vi "cblas zher2.vi"(0 "x":cdb[](array[numeric]), 1 "y":cdb[](array[numeric]), 2 "A":T2, 3 "alpha":cdb=1.0+0.0i, 5 "order":T3=101 items=["CblasRowMajor"=101, "CblasColMajor"=102], 7 "uplo":T1=121 items=["CblasUpper"=121, "CblasLower"=122], 8 "lda":i32, 10 "incx":i32=1, 11 "n":i32=-1, 12 "incy":i32=1) -> (14 "zher2":T2, 19 "error":i32)   [LabVIEW 2024, in "NI_AALBLAS.lvlib"]
uses:
  NI_AALBLAS.lvlib
  ComplexMatrix.ctl
  Order.ctl
  UpLo.ctl
  <resource>/lvblas.dll
  NI_Matrix.lvlib
panel:
  # "void cblas_zher2(order, uplo, n, *alpha, *x, incx, *y, incy, *A, lda)"
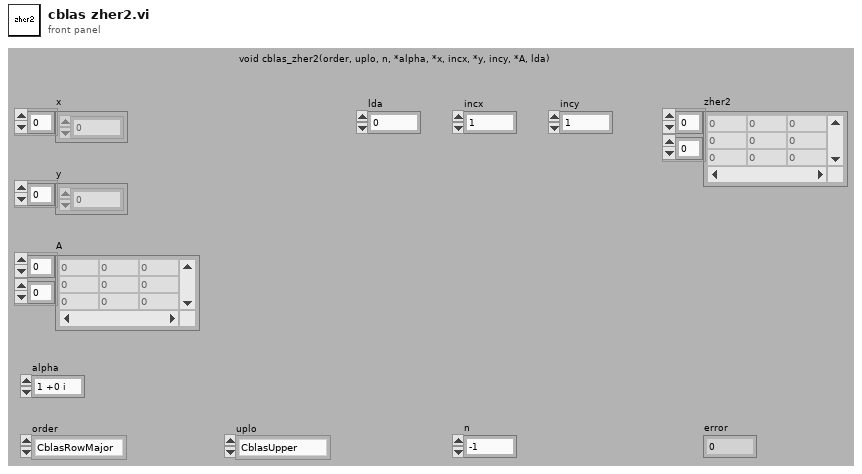
[diagram p1: front panel]
types:
  T1 = typedef "NI_AALBLAS.lvlib/UpLo.ctl" = i32
  T2 = typedef "NI_Matrix.lvlib/ComplexMatrix.ctl" = cdb[][]
  T3 = typedef "NI_AALBLAS.lvlib/Order.ctl" = i32
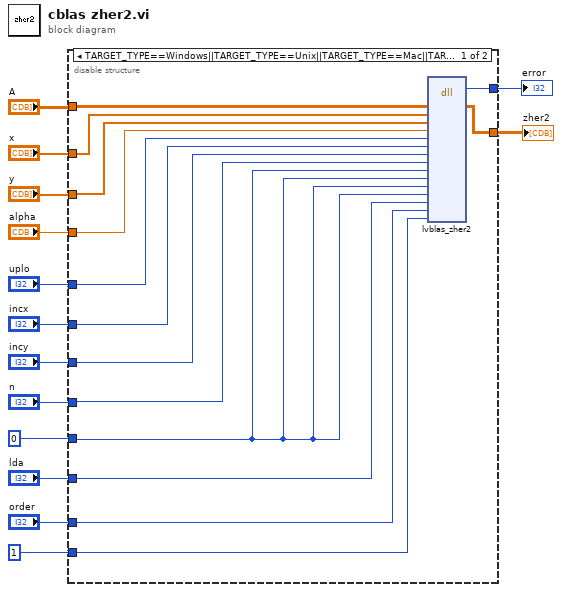
[diagram p0: block diagram]
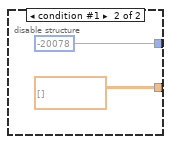
[diagram p2: hidden frame]
diagram:
  n1 = disable-structure shown="TARGET_TYPE==Windows||TARGET_TYPE==Unix||TARGET_TYPE==Mac||TARGET_TYPE==RT" {
    disable-tunnel: "x" -> [w25 _]
    disable-tunnel: "A" -> [w26 _]
    disable-tunnel: [w28 -20078 ("error")] -> w7
    disable-tunnel: 0 -> [w20 _]
    disable-tunnel: "lda" -> [w19 _]
    disable-tunnel: [w27 T2 [] ("Complex Matrix")] -> w8
    disable-tunnel: "uplo" -> [w22 _]
    disable-tunnel: "n" -> [w21 _]
    disable-tunnel: "alpha" -> [w23 _]
    disable-tunnel: "y" -> [w24 _]
    disable-tunnel: "order" -> [w18 _]
    disable-tunnel: "incx" -> [w17 _]
    disable-tunnel: "incy" -> [w16 _]
    disable-tunnel: 1 -> [w15 _]
    frame condition #0 (active) {
      n2 = dll-call lib="C:/Program Files (x86)/National Instruments/LabVIEW 2024/resource/lvblas.*" fn="lvblas_zher2" ("CBLAS.dll:MtrxxVectH")("a"=w26, "x"=w25, "y"=w24, "alpha"=w23, "uplo"=w22, "IncX"=w17, "IncY"=w16, "n"=w21, "startARow"=w20, "startACol"=w20, "startX"=w20, "startY"=w20, "lda"=w19, "order"=w18, "check"=w15) -> ("error"=w28:i32, "a"=w27:T2)  [unwired: 17 in, 2 out]
    }
    frame condition #1 {
    }
  }
  "error" <- w7
  "zher2" <- w8
